vi "State_Init_Script.vi"(8 "error in (no error)":errorcluster, 10 "Commands":T1[](array[typedef]), 11 "launcher in":refnum<class "launcher.lvclass">) -> (0 "error out":errorcluster, 2 "Debug Message":string, 3 "launcher out":refnum<class "launcher.lvclass">)   [LabVIEW 2021, in "launcher.lvclass"]
uses:
  launcher.lvclass
  <userlib>/S2 Labs/Queued State Machine/TypeDefs/Queue Message.ctl
  <userlib>/S2 Labs/Queued State Machine/TypeDefs/States.ctl
  <userlib>/S2 Labs/Module Framework/Modules/Base/Module.lvclass
  <userlib>/S2 Labs/Queued State Machine/QSM.lvclass
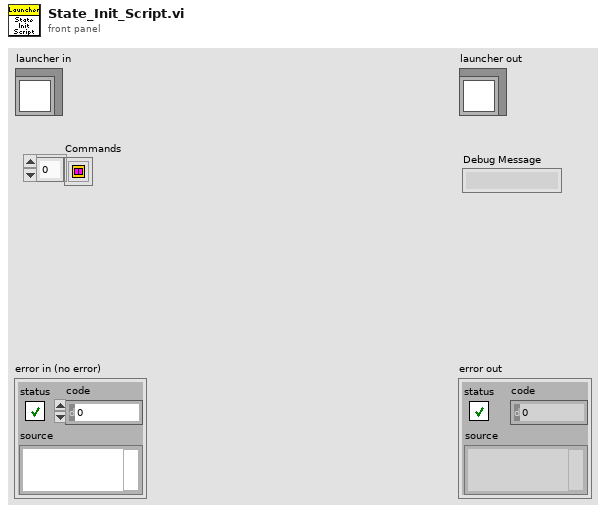
[diagram p1: front panel]
types:
  T1 = typedef "QSM.lvclass/Queue Message.ctl" = cluster{"State":T2, "Command":string, "Parameter":variant}
  T2 = typedef "QSM.lvclass/States.ctl" = enum16{"Waiting", "Init", "ExecCMD", "Read Config", "Write Config", "Launch", "Connect", "Recovery", "Clean Up", "Exit"}
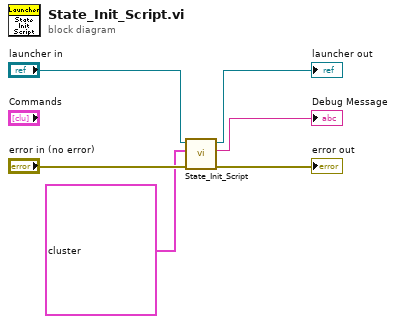
[diagram p0: block diagram]
diagram:
  n1 = call-parent "State_Init_Script.vi"("error in (no error)"="error in (no error)", "Commands"=T1[] [{"State"=enum."Launch", "Command"="FPGA", "Parameter"=variant}, {"State"=enum."Launch", "Command"="Module", "Parameter"=variant}], "Module in"="launcher in") -> ("error out"=→"error out":errorcluster, "Debug Message"=→"Debug Message":string, "Module out"=→"launcher out":refnum<class "launcher.lvclass">)  [unwired: 6 in]
